vi "ParseVectorFile.NewFileAsynchronous.vi"(8 "error in (no error)":errorcluster, 10 "NewFile":T1, 11 "ParseVectorFile":refnum<class "ParseVectorFile.lvclass">) -> (0 "error out":errorcluster, 3 "ParseVectorFile out":refnum<class "ParseVectorFile.lvclass">)   [LabVIEW 2019, in "ParseVectorFile.lvclass"]
doc: "---------------------------------------------------------------\nJKI State Machine Objects™\nhttp://jki.net/state-machine-objects/\nCopyright (C) 2005-2015, JKI <info@jki.net>\nALL RIGHTS RESERVEDJKI State Machine Objects (SMO) 1.0.0.4\nJKI - JKI\nCopyright (c) 2015, JKI"
uses:
  ParseVectorFile.lvclass
  Typedefs/PrivateEvents--ParseVectorFile.NewFile.ctl
  ParseVectorFile.lvclass/ParseVectorFile.ctl
panel:
  # "For instructions on how to use the JKI State Machine Objects, examples and video tutorials, visit:\nhttp://jki.net/state-machine-objects/\n\nJKI State Machine Objects™\nhttp://jki.net/state-machine-objects/\nCopyright (C) 2005-2015, JKI <info@jki.net>\nALL RIGHTS RESERVED"
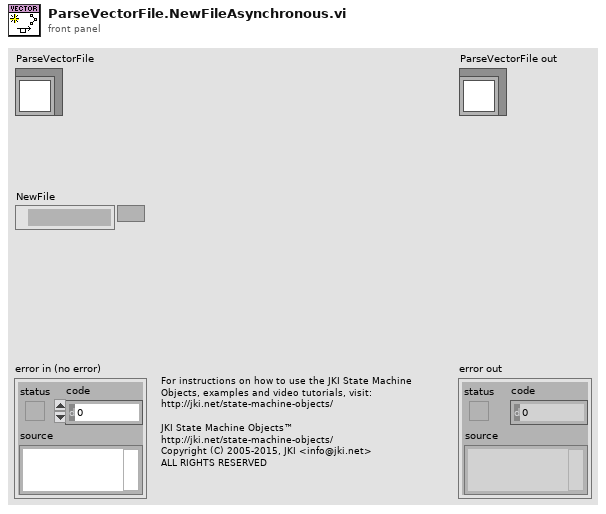
[diagram p1: front panel]
types:
  T1 = typedef "ParseVectorFile.lvclass/PrivateEvents--ParseVectorFile.NewFile.ctl" = path
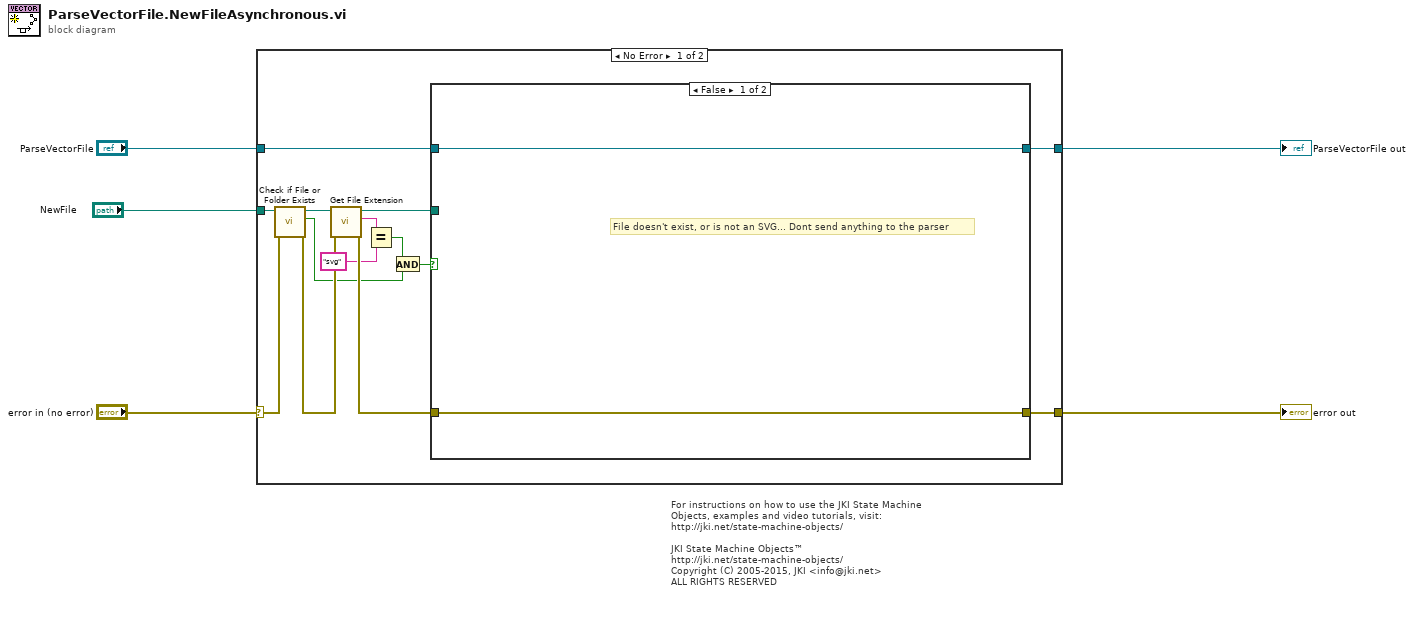
[diagram p0: block diagram]
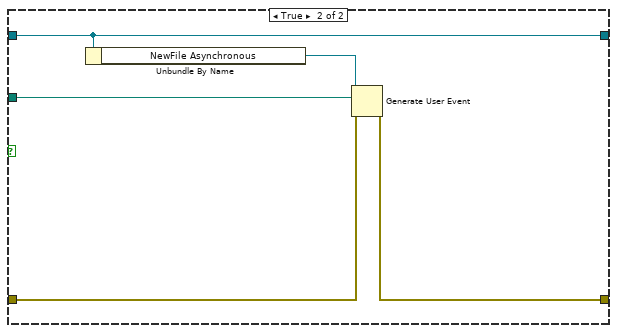
[diagram p2: hidden frame]
diagram:
  # "For instructions on how to use the JKI State Machine Objects, examples and video tutorials, visit:\nhttp://jki.net/state-machine-objects/\n\nJKI State Machine Objects™\nhttp://jki.net/state-machine-objects/\nCopyright (C) 2005-2015, JKI <info@jki.net>\nALL RIGHTS RESERVED"
  n1 = case shown="No Error" "error in (no error)" {
    selector: "error in (no error)" -> [w15 w28]
    tunnel: [w19 w28] -> w4
    tunnel: [w17 w27] -> w5
    tunnel: "ParseVectorFile" -> [w18 w27]
    tunnel: "NewFile" -> [w16 _]
    frame No Error {
      n2 = call <vilib>:"Check if File or Folder Exists.vi"("error in (no error)"=w15, "path"=w16) -> ("error out"=w12:errorcluster, "file or folder exists?"=w7:bool, "dup path"=w14:path)  [unwired: 7 in]
      n3 = call <vilib>:"Get File Extension.vi"("error in (no error)"=w12, "file"=w14) -> ("error out"=w11:errorcluster, "lowercase file extension"=w10:string, "dup file"=w13:path)  [unwired: 5 in, 2 out]
      n4 = Equal?(x=w10, y="svg") -> (x = y?=w8:bool)
      n5 = And(x=w8, y=w7) -> (x .and. y?=w6:bool)
      n6 = case shown="False" w6 {
        tunnel: w11 -> [w20 w26]
        tunnel: w13 -> [_ w25]
        tunnel: [w20 w24] -> w19
        tunnel: w18 -> [w21 w22]
        tunnel: [w21 w22] -> w17
        frame False {
          # "File doesn't exist, or is not an SVG... Dont send anything to the parser"
        }
        frame True {
          n7 = Unbundle By Name(w22) -> ("NewFile Asynchronous"=w23:refnum<user-event>)
          n8 = Generate User Event(user event=w23, event data cluster=w25, error in=w26) -> (error out=w24:errorcluster)  [unwired: 1 in, 1 out]
        }
      }
    }
    frame Error {
    }
  }
  "error out" <- w4
  "ParseVectorFile out" <- w5
